vi "Disconnect_Voltage_Reference_from_UUT_set_PS1_15V.vi"(3 "error in":errorcluster) -> (10 "error out":errorcluster)   [LabVIEW 2015]
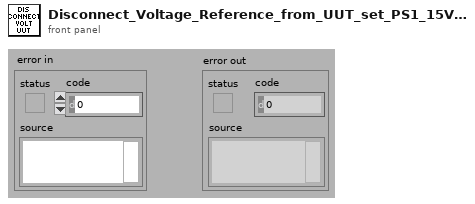
[diagram p1: front panel]
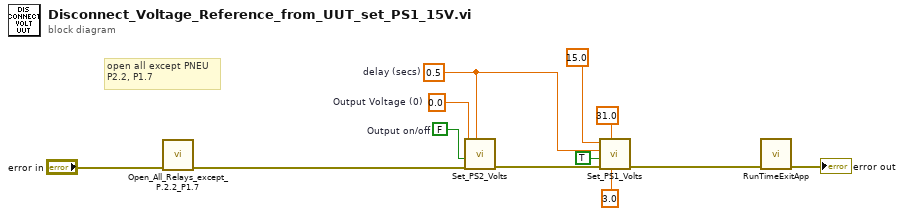
[diagram p0: block diagram]
diagram:
  w8 = FALSE  # Output on/off
  w4 = 0.5  # delay (secs)
  w11 = 0.0  # Output Voltage (0)
  # "open all except PNEU\nP2.2, P1.7"
  n1 = call "Open_All_Relays_except_P.2.2_P1.7.vi"("error in"="error in") -> ("error out"=w9:errorcluster)  [unwired: 8 in]
  n2 = call "Set_PS2_Volts.vi"("delay (secs)"=w4, "error in"=w9, "Output on/off"=w8, "Output Voltage"=w11) -> ("error out"=w7:errorcluster)  [unwired: 5 in, 2 out]
  n3 = call "Set_PS1_Volts.vi"("Current Limit (0)"=3.0, "Maximum Output Voltage (31)"=31.0, "error in"=w7, "Output on/off"=TRUE, "delay (secs)"=w4, "Output Voltage"=15.0) -> ("error out"=w6:errorcluster)  [unwired: 3 in, 2 out]
  n4 = call "RunTimeExitApp.vi"("error in (no error)"=w6) -> ("error out"=→"error out":errorcluster)  [unwired: 10 in]
